vi "Read Wfm Data.vi"(8 "error in (no error)":errorcluster, 11 "Async State Vars in":T1) -> (0 "error out":errorcluster, 1 "samples read":i32, 3 "Async State Vars out":T1, 4 "Wfm timed out?":bool)   [LabVIEW 2020, in "Waveform-Processing-Custom-Device Engine.lvlib"]
uses:
  Waveform-Processing-Custom-Device Engine.lvlib
  <vilib>/NI VeriStand/Custom Device Waveform API/NI_VS Custom Device Waveform API.lvlib
  <vilib>/NI VeriStand/Custom Device Waveform API/Single Waveform Read (DBL)/NI VeriStand - Read Single Waveform (DBL).vi
  <vilib>/NI VeriStand/Custom Device Waveform API/Single Waveform Read (DBL)/Single Waveform Read (DBL).lvclass
  <userlib>/Circular Buffer/Instance VIs/Circular Buffer(2D DBL).vi
  <userlib>/Circular Buffer/Controls/Circular Buffer Operations.ctl
  Types/AsyncStateVariables.ctl
  <vilib>/NI VeriStand/Custom Device Waveform API/Single Waveform Write (DBL)/Single Waveform Write (DBL).lvclass
  <vilib>/NI VeriStand/Custom Device API/Waveform Data Reference.ctl
  <vilib>/NI VeriStand/Custom Device API/Custom Device API.lvlib
  <vilib>/NI/NIVS Inline Async API/_Data Access Engine/Access Type Classes/Read/Read.lvclass
  <vilib>/NI/NIVS Inline Async API/_Data Access Engine/Data Access Engine/Types/Read.DVR.ctl
  <vilib>/NI/NIVS Inline Async API/_Data Access Engine/Data Access Engine/Data Access Engine.lvclass
  <vilib>/NI/NIVS Inline Async API/_Data Access Engine/Access Type Classes/Write/Write.lvclass
  <vilib>/NI/NIVS Inline Async API/_Data Access Engine/Data Access Engine/Types/Write.DVR.ctl
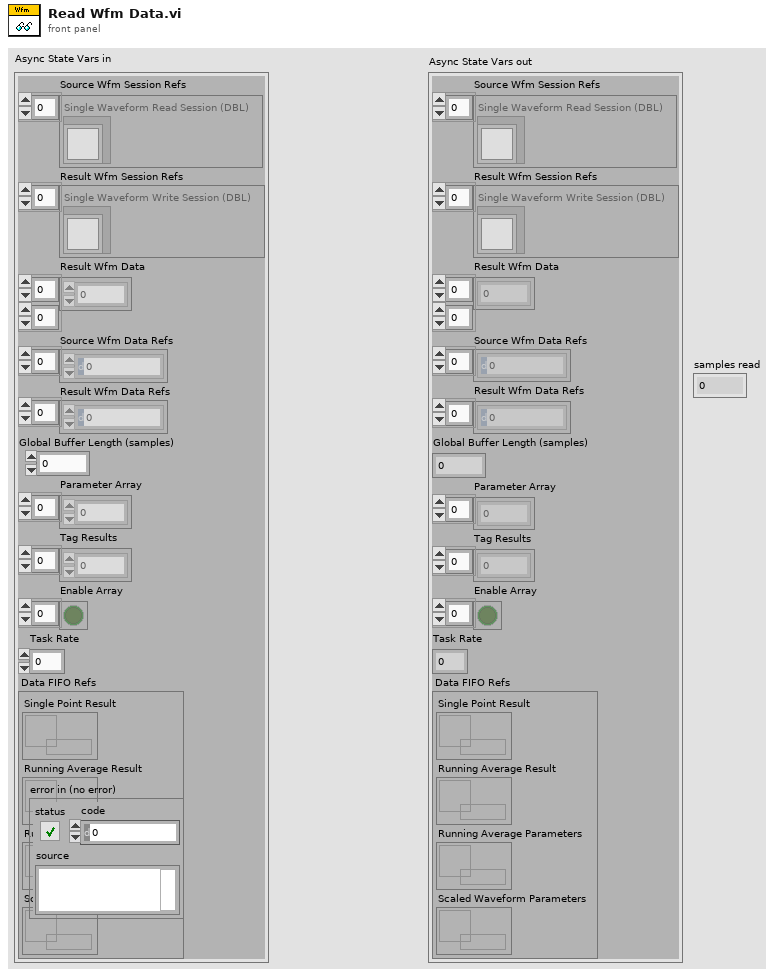
[diagram p1: front panel]
types:
  T1 = typedef "Waveform-Processing-Custom-Device Engine.lvlib/AsyncStateVariables.ctl" = cluster{"Source Wfm Session Refs":refnum<class "Single Waveform Read (DBL).lvclass">[], "Result Wfm Session Refs":refnum<class "Single Waveform Write (DBL).lvclass">[], "Result Wfm Data":dbl[][], "Source Wfm Data Refs":T2[], "Result Wfm Data Refs":T2[], "Global Buffer Length (samples)":dbl, "Parameter Array":dbl[], "Tag Results":dbl[], "Enable Array":bool[], "Task Rate":dbl, "Data FIFO Refs":cluster{"Single Point Result":T3, "Running Average Result":T3, "Running Average Parameters":T4, "Scaled Waveform Parameters":T4}}
  T2 = typedef "Custom Device API.lvlib/Waveform Data Reference.ctl" = i32
  T3 = typedef "Data Access Engine.lvlib/Data Access Engine.lvclass/Write.DVR.ctl" = refnum<data-value>
  T4 = typedef "Data Access Engine.lvlib/Data Access Engine.lvclass/Read.DVR.ctl" = refnum<data-value>
  T5 = typedef "Circular Buffer.lvlib/Circular Buffer Operations.ctl" = enum16{"Initialize", "Get Backlog", "Write", "Read (continuous)", "Read (most recent)"}
  T6 = typedef "NI_VS Custom Device Waveform API.lvlib/Waveform properties.ctl" = cluster{"Data reference":T2, "t0 at start":timestamp, "dt":dbl, "offset from start (samples)":u64}
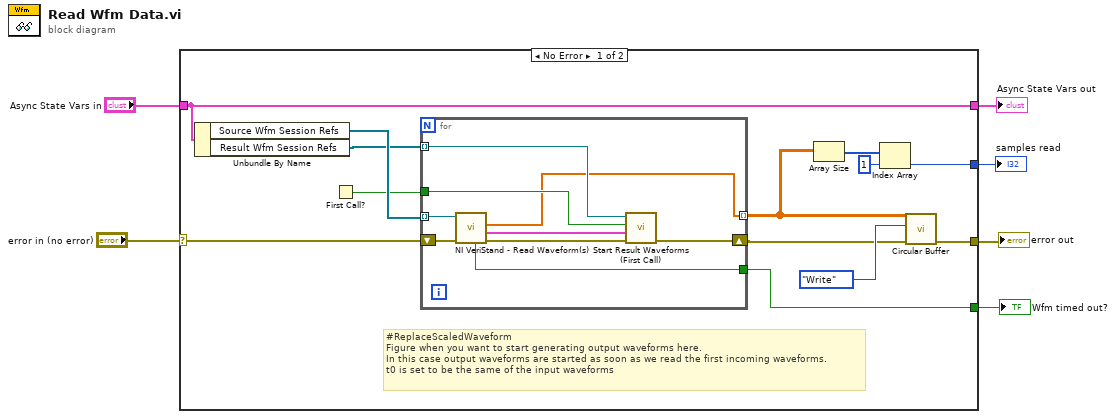
[diagram p0: block diagram]
diagram:
  n1 = case shown="No Error" "error in (no error)" {
    selector: "error in (no error)" -> [w16 w29]
    tunnel: [w17 w29] -> w6
    tunnel: "Async State Vars in" -> [w15 w30]
    tunnel: [w15 w30] -> w3
    tunnel: [w14 _] -> w2
    tunnel: [w8 _] -> w1
    frame No Error {
      # "#ReplaceScaledWaveform \nFigure when you want to start generating output waveforms here.\nIn this case output waveforms are started as soon as we read the first incoming waveforms.\nt0 is set to be the same of the input waveforms"
      n2 = Unbundle By Name(w15) -> ("Source Wfm Session Refs"=w19:refnum<class "Single Waveform Read (DBL).lvclass">[], "Result Wfm Session Refs"=w12:refnum<class "Single Waveform Write (DBL).lvclass">[])
      n3 = First Call?() -> (First Call?: T/F=w13:bool)
      n4 = for {
        tunnel: [w21] -> w11 mode=indexing
        tunnel: [w27] -> w14
        tunnel: w19 -> [w26] mode=indexing
        tunnel: w13 -> [w22]
        tunnel: w12 -> [w23] mode=indexing
        shift-right: [w20] -> w7
        shift-left: w16 -> [w28]
        n5 = call-poly <vilib>:"NI VeriStand - Read Waveform(s).vi"("error in (no error)"=w28, "Single Waveform Read Session (DBL) in"=w26) -> ("error out"=w25:errorcluster, "Properties"=w24:T6, "Data"=w21:dbl[], "timed out?"=w27:bool)  [unwired: 5 in, 1 out]
        n6 = call "Start Result Waveforms (First Call).vi"("error in (no error)"=w25, "Properties"=w24, "First Call?"=w22, "Result Wfm Session Ref"=w23) -> ("error out"=w20:errorcluster)  [unwired: 7 in]
      }
      n7 = Array Size(array=w11) -> (size(s)=w10:i32[])
      n8 = Index Array(array=w10, index=1) -> (element=w8:i32)
      n9 = call-poly <userlib>:"Circular Buffer.vi"("error in (no error)"=w7, "Operation"=Circular_Buffer_Operations."Write", "Data In"=w11) -> ("error out"=w17:errorcluster)  [unwired: 5 in, 3 out]
    }
    frame Error {
    }
  }
  "error out" <- w6
  "Wfm timed out?" <- w2
  "Async State Vars out" <- w3
  "samples read" <- w1
